vi "Read IMAQ Image.vi"(0 "image in":refnum<class "MSC Image.lvclass">, 1 "IMAQ Image":T1, 5 "error in (no error)":errorcluster) -> (14 "image out":refnum<class "MSC Image.lvclass">, 15 "IMAQ Image out":T1, 19 "error out":errorcluster)   [LabVIEW 2016]
doc: "Converts an IMAQ Image to a MSC Image. \n\nThe IMAQ Image is still in memory ! Use IMAQ Dispose to clear it."
uses:
  MSC Image.lvclass
  <vilib>/vision/Image Controls.llb/IMAQ Image.ctl
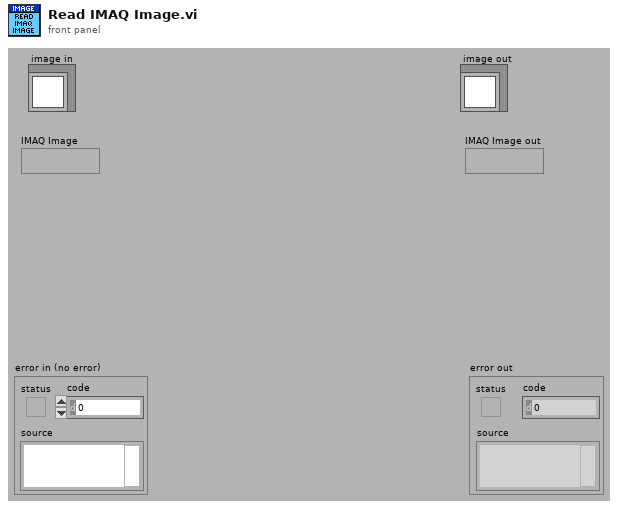
[diagram p1: front panel]
types:
  T1 = typedef "IMAQ Image.ctl" = refnum<image>
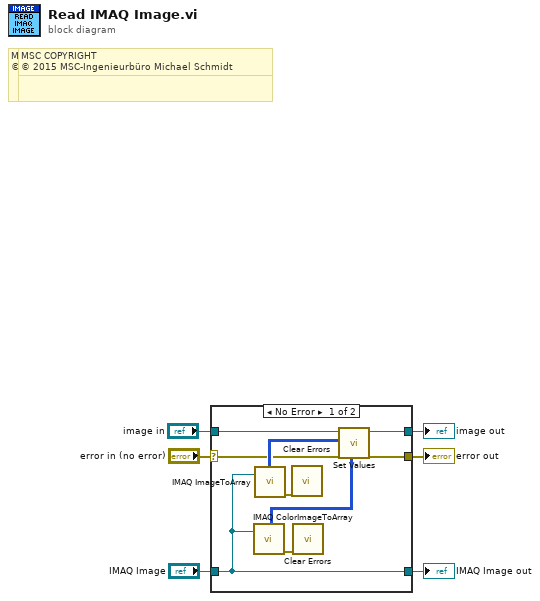
[diagram p0: block diagram]
diagram:
  # "MSC COPYRIGHT\n© 2016 MSC-Ingenieurbüro Michael Schmidt"
  # "MSC COPYRIGHT\n© 2016 MSC-Ingenieurbüro Michael Schmidt"
  # "MSC COPYRIGHT\n© 2015 MSC-Ingenieurbüro Michael Schmidt"
  # "MSC COPYRIGHT\n© 2015 MSC-Ingenieurbüro Michael Schmidt"
  n1 = case shown="No Error" "error in (no error)" {
    selector: "error in (no error)" -> [w7 w20]
    tunnel: [w17 w20] -> w5
    tunnel: [w12 w19] -> w3
    tunnel: "image in" -> [w13 w19]
    tunnel: "IMAQ Image" -> [w10 w18]
    tunnel: [w10 w18] -> w1
    frame No Error {
      n2 = call "IMAQ ColorImageToArray"("Image"=w10) -> ("Image Pixels (U32)"=w11:u32[][], "error out"=w9:errorcluster)  [unwired: 3 in, 1 out]
      n3 = call "IMAQ ImageToArray"("Image"=w10) -> ("Image Pixels (U16)"=w16:u16[][], "Image Pixels (Float)"=w15:sgl[][], "error out"=w8:errorcluster, "Image Pixels (U8)"=w14:u8[][])  [unwired: 3 in, 1 out]
      n4 = call <vilib>:"Clear Errors.vi"("error in (no error)"=w8) -> ()  [unwired: 5 in, 2 out]
      n5 = call <vilib>:"Clear Errors.vi"("error in (no error)"=w9) -> ()  [unwired: 5 in, 2 out]
      n6 = call-dynamic "Set Values.vi"("image in"=w13, "imageData U8"=w14, "imageData U16"=w16, "imageData Single"=w15, "error in (no error)"=w7, "imageData BGR"=w11) -> ("image out"=w12:refnum<class "MSC Image.lvclass">, "error out"=w17:errorcluster)  [unwired: 12 in]
    }
    frame Error {
    }
  }
  "error out" <- w5
  "image out" <- w3
  "IMAQ Image out" <- w1
